vi "RVC Rotation Matrix not Commutative.vi"() -> ()   [LabVIEW 2013]
uses:
  <vilib>/Analysis/baseanly.llb/Real A x B.vi
  <vilib>/Analysis/_algsub.llb/Vector Norm.vi
  <vilib>/Analysis/_algsub.llb/Real Vector Norm.vi
  <vilib>/Analysis/baseanly.llb/Outer Product.vi
  <vilib>/Analysis/baseanly.llb/Real Outer Product.vi
  <vilib>/robotics/Kinematics/Create Lie Group Matrix.vi
  <vilib>/Analysis/Matrix/Numeric/Multiply/Multiply - RM,RM.vi
  <vilib>/Analysis/7linalg.llb/Create Special Matrix.vi
  <vilib>/Analysis/7linalg.llb/Create Special Real Matrix.vi
  <vilib>/Analysis/Matrix/Numeric/Multiply/Multiply - RM,R.vi
  <vilib>/Analysis/Matrix/Numeric/Multiply/Multiply - R,RM.vi
  <vilib>/Analysis/Matrix/Numeric/Add/Add.vi
  <vilib>/Analysis/Matrix/Numeric/Add/Add - RM,RM.vi
  <vilib>/robotics/Kinematics/NI_Kinematics.lvlib
  <vilib>/Analysis/NI_AALBase.lvlib
  <vilib>/Analysis/Matrix/NI_Matrix.lvlib
panel:
  out "transformation matrix 3":picture
  out "3D Picture 4":refnum<vi>(3d-picture)
  out "transformation matrix 2":picture
  out "3D Picture 3":refnum<vi>(3d-picture)
  out "3D Picture 2":refnum<vi>(3d-picture)
  out "3D Picture":refnum<vi>(3d-picture)
  out "commutative transformation matrix":picture
  out "transformation matrix":picture
  # "is different than"
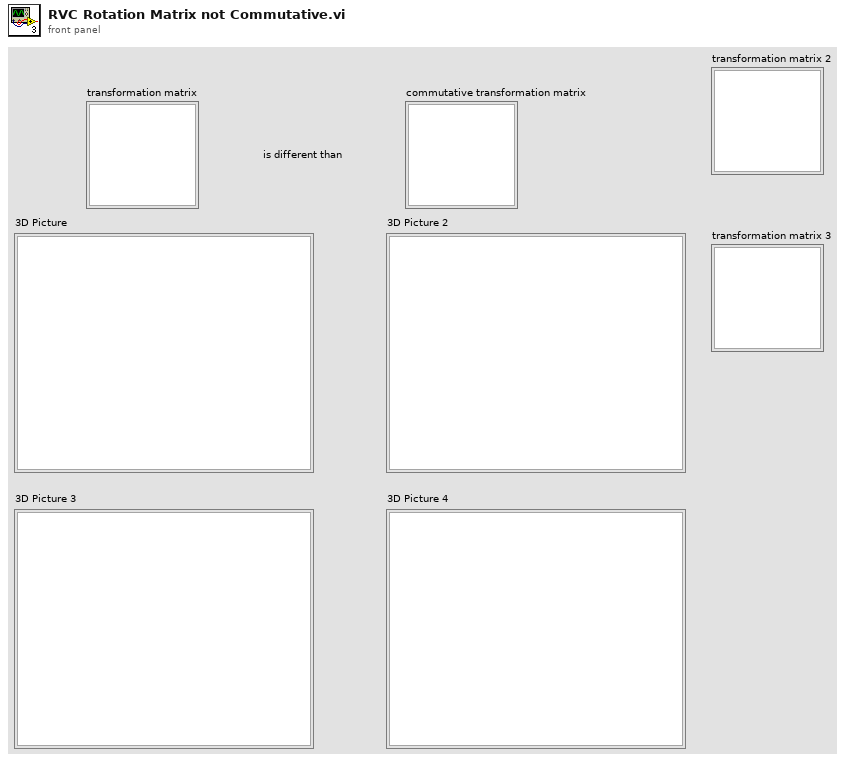
[diagram p1: front panel]
types:
  T1 = typedef "NI_Matrix.lvlib/RealMatrix.ctl" = dbl[][]
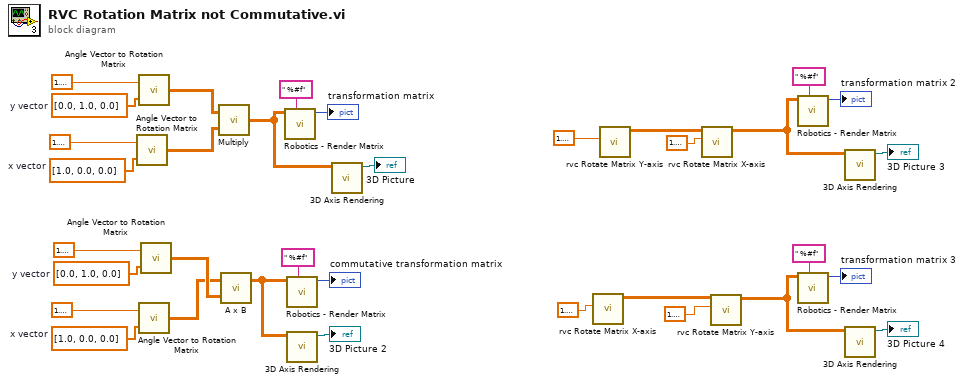
[diagram p0: block diagram]
diagram:
  w25 = dbl[] [0.0, 1.0, 0.0]  # y vector
  w20 = dbl[] [1.0, 0.0, 0.0]  # x vector
  w28 = dbl[] [0.0, 1.0, 0.0]  # y vector
  w33 = dbl[] [1.0, 0.0, 0.0]  # x vector
  n1 = call <vilib>:"Angle Vector to Rotation Matrix.vi"("vector"=w33, "angle"=1.5707963267948966) -> ("rotation matrix"=w30:T1)
  n2 = call <vilib>:"Angle Vector to Rotation Matrix.vi"("vector"=w28, "angle"=1.5707963267948966) -> ("rotation matrix"=w27:T1)
  n3 = call <vilib>:"Angle Vector to Rotation Matrix.vi"("vector"=w20, "angle"=1.5707963267948966) -> ("rotation matrix"=w23:T1)
  n4 = call <vilib>:"Angle Vector to Rotation Matrix.vi"("vector"=w25, "angle"=1.5707963267948966) -> ("rotation matrix"=w26:T1)
  n5 = call-poly <vilib>:"Multiply.vi"("Real Matrix B"=w30, "Real Matrix A"=w27) -> ("A * B"=w15:T1)
  n6 = call-poly <vilib>:"A x B.vi"("B"=w26, "A"=w23) -> ("A x B"=w16:T1)  [unwired: 1 out]
  n7 = call "Robotics - Render Matrix.vi"("format string"=" %#f", "A"=w15) -> ("picture out"=→"transformation matrix":picture)  [unwired: 9 in]
  n8 = call "Robotics - Render Matrix.vi"("format string"=" %#f", "A"=w16) -> ("picture out"=→"commutative transformation matrix":picture)  [unwired: 9 in]
  n9 = call "3D Axis Rendering.vi"("rotation matrix"=w16) -> ("SceneNode out"=→"3D Picture 2":refnum<vi>)  [unwired: 9 in, 1 out]
  n10 = call "3D Axis Rendering.vi"("rotation matrix"=w15) -> ("SceneNode out"=→"3D Picture":refnum<vi>)  [unwired: 9 in, 1 out]
  n11 = call "rvc Rotate Matrix X-axis.vi"("angle"=1.5707963267948966) -> ("rotation matrix"=w2:T1)  [unwired: 10 in]
  n12 = call "rvc Rotate Matrix Y-axis.vi"("angle"=1.5707963267948966) -> ("rotation matrix"=w13:T1)  [unwired: 10 in]
  n13 = call "rvc Rotate Matrix X-axis.vi"("angle"=1.5707963267948966, "rotation matrix in"=w13) -> ("rotation matrix"=w9:T1)  [unwired: 9 in]
  n14 = call "rvc Rotate Matrix Y-axis.vi"("angle"=1.5707963267948966, "rotation matrix in"=w2) -> ("rotation matrix"=w1:T1)  [unwired: 9 in]
  n15 = call "Robotics - Render Matrix.vi"("format string"=" %#f", "A"=w9) -> ("picture out"=→"transformation matrix 2":picture)  [unwired: 9 in]
  n16 = call "Robotics - Render Matrix.vi"("format string"=" %#f", "A"=w1) -> ("picture out"=→"transformation matrix 3":picture)  [unwired: 9 in]
  n17 = call "3D Axis Rendering.vi"("rotation matrix"=w9) -> ("SceneNode out"=→"3D Picture 3":refnum<vi>)  [unwired: 9 in, 1 out]
  n18 = call "3D Axis Rendering.vi"("rotation matrix"=w1) -> ("SceneNode out"=→"3D Picture 4":refnum<vi>)  [unwired: 9 in, 1 out]
